vi "Connect Subpanel to Manager.vi"(8 "error in (no error)":errorcluster, 10 "Manager Port":u16=15882, 11 "CIF_UI in":refnum<class "CIF_UI.lvclass">) -> (3 "CIF_UI out":refnum<class "CIF_UI.lvclass">)   [LabVIEW 2021, in "CIF_UI.lvclass"]
uses:
  CIF_UI.lvclass
  CIF_UI.lvclass/CIF_UI.ctl
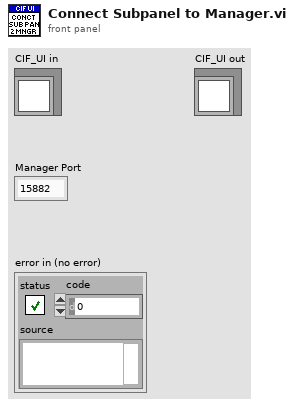
[diagram p1: front panel]
types:
  T1 = typedef "grpc-lvsupport-release.lvlib/grpcId.ctl" = u64
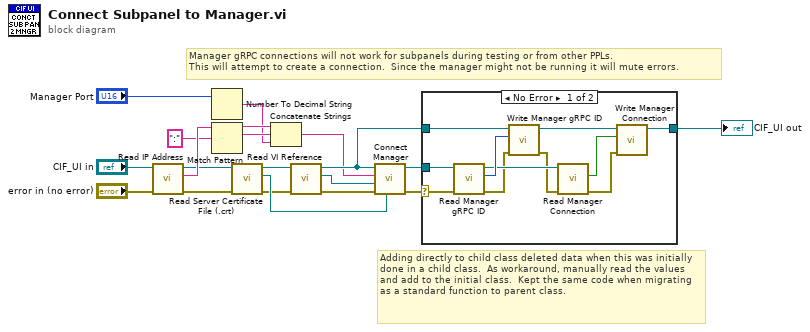
[diagram p0: block diagram]
diagram:
  # "Adding directly to child class deleted data when this was initially done in a child class.  As workaround, manually read the values and add to the initial class.  Kept the same code when migrating as a standard function to parent class."
  # "Manager gRPC connections will not work for subpanels during testing or from other PPLs.  \nThis will attempt to create a connection.  Since the manager might not be running it will mute errors."
  n1 = call "Read IP Address.vi"("error in (no error)"="error in (no error)", "CIF_UI in"="CIF_UI in") -> ("error out"=w15:errorcluster, "IP address"=w19:string, "CIF_UI out"=w16:refnum<class "CIF_UI.lvclass">)  [unwired: 7 in]
  n2 = Number To Decimal String(number="Manager Port") -> (decimal integer string=w1:string)  [unwired: 1 in]
  n3 = Match Pattern(string=w19, regular expression=":") -> (before substring=w3:string, match substring=w2:string)  [unwired: 1 in, 2 out]
  n4 = call "Read Server Certificate File (.crt).vi"("error in (no error)"=w15, "CIF_UI in"=w16) -> ("error out"=w13:errorcluster, "Server Certificate File (.crt)"=w17:path, "CIF_UI out"=w14:refnum<class "CIF_UI.lvclass">)  [unwired: 7 in]
  n5 = Concatenate Strings(w3, w2, w1) -> (w4:string)
  n6 = call "Read VI Reference.vi"("error in (no error)"=w13, "CIF_UI in"=w14) -> ("error out"=w12:errorcluster, "VI Reference"=w11:refnum<vi>, "CIF_UI out"=w9:refnum<class "CIF_UI.lvclass">)  [unwired: 7 in]
  n7 = call "Connect Manager.vi"("Server Certificate File (.crt)"=w17, "error in (no error)"=w12, "VI Reference"=w11, "Address"=w4, "CIF_UI in"=w9) -> ("error out"=w10:errorcluster, "CIF_UI out"=w8:refnum<class "CIF_UI.lvclass">)  [unwired: 5 in]
  n8 = case shown="No Error" w10 {
    selector: w10 -> [w30 _]
    tunnel: w8 -> [w31 _]
    tunnel: [w21 w32] -> w6
    tunnel: w9 -> [w29 w32]
    frame No Error {
      n9 = call "Read Manager gRPC ID.vi"("error in (no error)"=w30, "CIF_UI in"=w31) -> ("error out"=w26:errorcluster, "Manager gRPCid"=w28:T1, "CIF_UI out"=w27:refnum<class "CIF_UI.lvclass">)  [unwired: 7 in]
      n10 = call "Write Manager gRPC ID.vi"("error in (no error)"=w26, "gRPCid"=w28, "CIF_UI in"=w29) -> ("error out"=w25:errorcluster, "CIF_UI out"=w24:refnum<class "CIF_UI.lvclass">)  [unwired: 7 in]
      n11 = call "Read Manager Connection.vi"("error in (no error)"=w25, "CIF_UI in"=w27) -> ("error out"=w23:errorcluster, "Manager Connection"=w22:bool)  [unwired: 7 in, 1 out]
      n12 = call "Write Manager Connection.vi"("error in (no error)"=w23, "Manager Connection"=w22, "CIF_UI in"=w24) -> ("CIF_UI out"=w21:refnum<class "CIF_UI.lvclass">)  [unwired: 7 in, 1 out]
    }
    frame Error {
    }
  }
  "CIF_UI out" <- w6
